vi "SW_Draw_mouse_DAQmx.vi"(0 "Image In":T1, 1 "Size of the image (480x480)":T3={"Numeric Control"=480.0, "Numeric Control"=480.0}, 5 "Pixels per mm":dbl=2.0, 7 "Mouse position":T2, 9 "Trace length, samples":u16=20 max=1000 step=1, 11 "Bright mouse lineout":bool=TRUE, 12 "Colors array input":u32[](array[colorbox]), 13 "Rainbow colors":bool=TRUE) -> (4 "Image Out":T1)   [LabVIEW 2018]
uses:
  <vilib>/vision/Image Controls.llb/IMAQ Image.ctl
  <vilib>/Utility/miscctls.llb/LVBoundsTypeDef.ctl
panel:
  in  "Experiment Diagram":T1(plugin-control)=refnum
  out "Time per draw":dbl
  in  "Trace color 2":u32(colorbox)
  in  "Trace color":u32(colorbox)=16757314
  in  "Mouse lineout color":u32(colorbox)=16775210
  in  "Iris size factor":dbl=0.05000000000000001 min=0.01 max=0.22 step=0.005 format="%#_13g"
  in  "Eye size factor":dbl=0.07000000000000002 min=0.02 max=0.24 step=0.01 format="%#_13g"
  out "Mouse abs. coordinates, pix":T3={"Numeric Control"=240.0, "Numeric Control"=240.0}
  in  "Mouse color":u32(colorbox)=5460819
  in  "Mouse length, mm":dbl=40.0
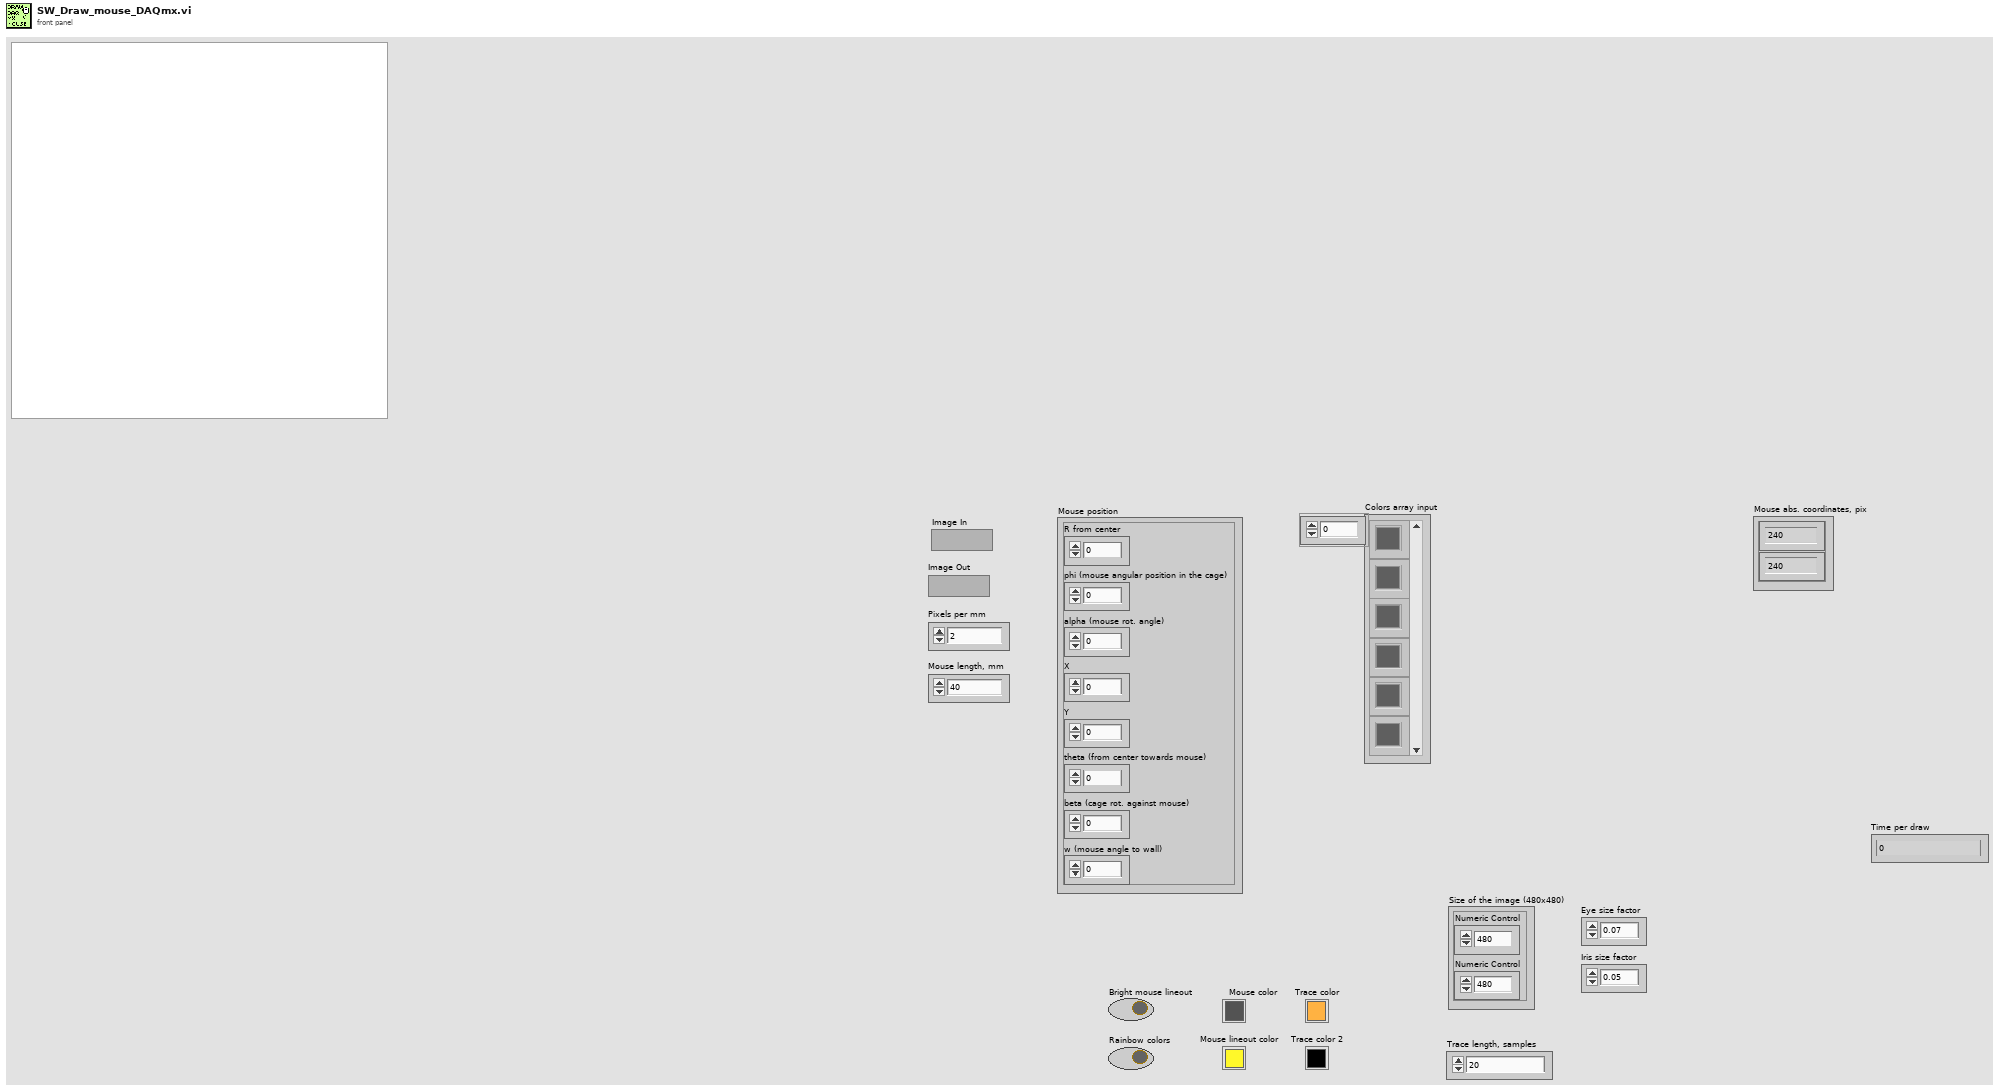
[diagram p1: front panel]
types:
  T1 = typedef "IMAQ Image.ctl" = refnum<image>
  T2 = cluster{"R from center":dbl, "phi (mouse angular position in the cage)":dbl, "alpha (mouse rot. angle)":sgl, "X":dbl, "Y":dbl, "theta (from center towards mouse)":dbl, "beta (cage rot. against mouse)":sgl, "w (mouse angle to wall)":dbl}
  T3 = cluster{"Numeric Control":dbl, "Numeric Control":dbl}
  T4 = cluster{"Width":u16, "Style":enum32{"Solid", "Dash", "Dot", "DashDot", "DashDotDot"}}
  T5 = typedef "LVBoundsTypeDef.ctl" = cluster{"Width":u32, "Height":u32}
  T6 = cluster{"Top":i32, "Left":i32, "Bottom":i32, "Right":i32}
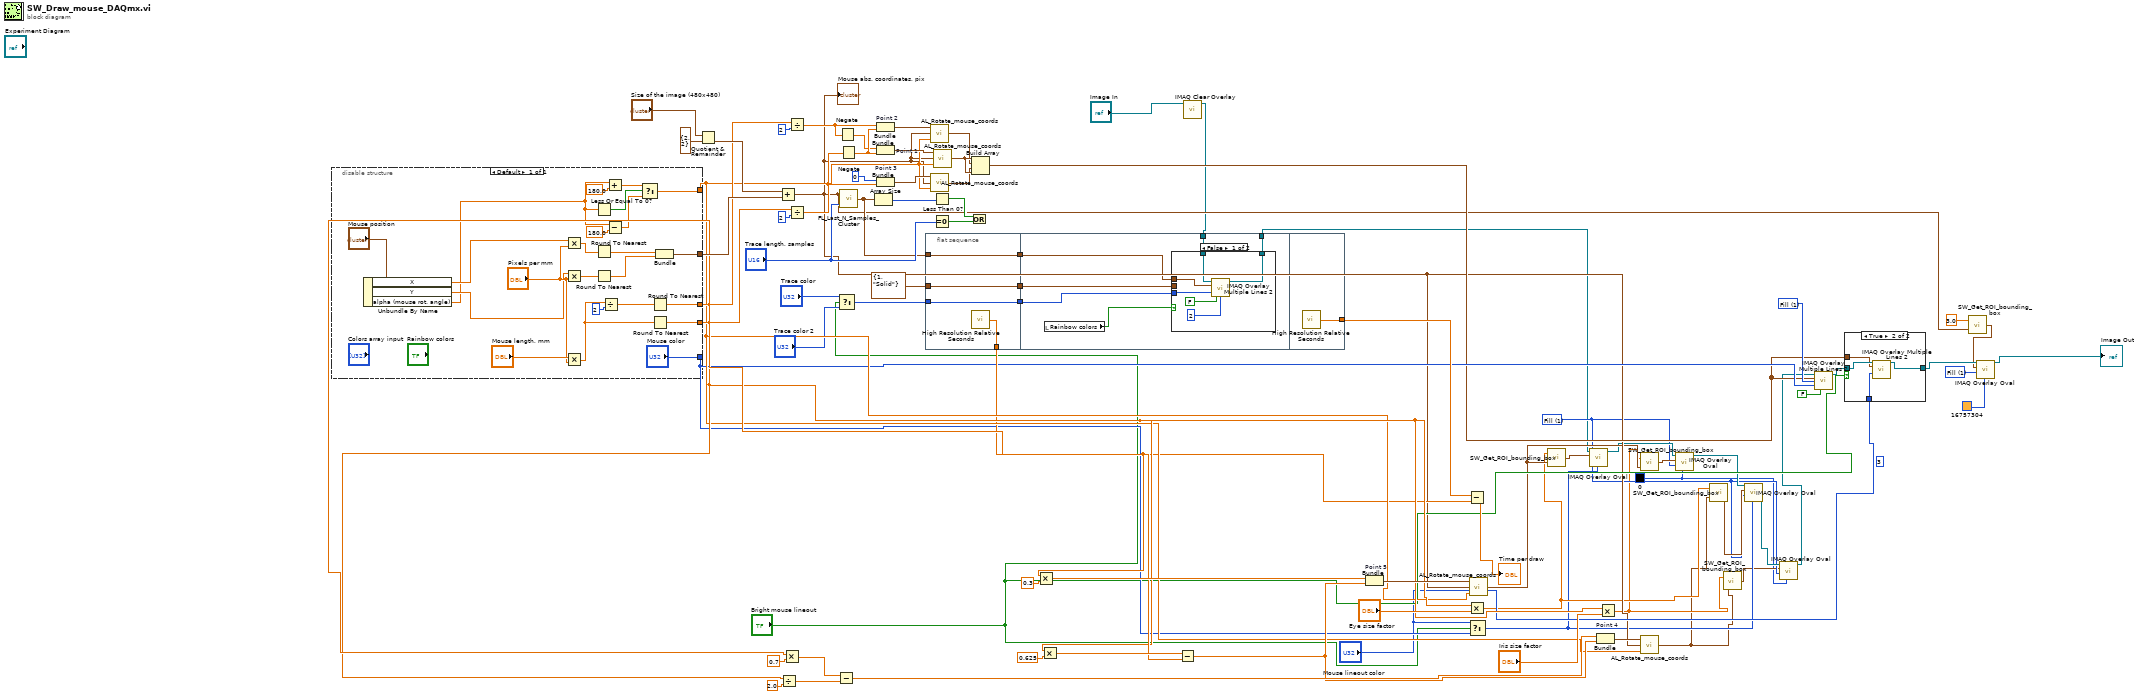
[diagram p0: block diagram]
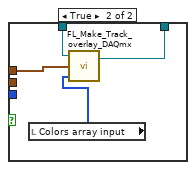
[diagram p3: hidden frame]
diagram:
  w4 = u32 0 ("Color")
  w8 = u32 1 items=["Frame", "Fill"] ("Drawing Mode (Frame)")
  w22 = u32 1 items=["Frame", "Fill"] ("Drawing Mode (Frame)")
  w32 = u32 1 items=["Frame", "Fill"] ("Drawing Mode (Frame)")
  (unwired) i16 3 ("radius")
  n1 = disable-structure shown="Default" {
    disable-tunnel: ["Mouse color"] -> w31
    disable-tunnel: [w98] -> w53
    disable-tunnel: [w100] -> w52
    disable-tunnel: [w86] -> w50
    disable-tunnel: [w92] -> w65
    frame Enabled {
      n2 = Unbundle By Name("Mouse position") -> ("X"=w84:dbl, "Y"=w83:dbl, "alpha (mouse rot. angle)"=w82:sgl)
      n3 = Multiply(x=w84, y="Pixels per mm") -> (x*y=w97:dbl)
      n4 = Multiply(x=w83, y="Pixels per mm") -> (x*y=w96:dbl)
      n5 = Multiply(x="Mouse length, mm", y="Pixels per mm") -> (x*y=w101:dbl)
      n6 = Less Or Equal To 0?(x=w82) -> (x <= 0?=w91:bool)
      n7 = Round To Nearest(number=w97) -> (nearest integer value=w94:dbl)
      n8 = Round To Nearest(number=w96) -> (nearest integer value=w93:dbl)
      n9 = Divide(x=w101, y=2) -> (x/y=w99:dbl)
      n10 = Add(x=w82, y=sgl 180.0) -> (x+y=w88:sgl)
      n11 = Subtract(x=w82, y=sgl 180.0) -> (x-y=w90:sgl)
      n12 = Select(t=w88, s=w91, f=w90) -> (s? t:f=w86:sgl)
      n13 = Round To Nearest(number=w99) -> (nearest integer value=w98:dbl)
      n14 = Round To Nearest(number=w101) -> (nearest integer value=w100:dbl)
      n15 = Bundle(w94, w93) -> (w92:cluster{dbl, dbl})  [unwired: 1 in]
    }
  }
  n16 = Quotient & Remainder(x="Size of the image (480x480)", y=T5 {"Width"=2, "Height"=2}) -> (floor(x/y)=w64:cluster{dbl, dbl})  [unwired: 1 out]
  n17 = Add(x=w64, y=w65) -> (x+y=w21:cluster{dbl, dbl})
  "Mouse abs. coordinates, pix" <- w21
  n18 = Divide(x=w52, y=2.0) -> (x/y=w58:dbl)
  n19 = Multiply(x=w53, y=0.7) -> (x*y=w62:dbl)
  n20 = Divide(x=w53, y=u16 2) -> (x/y=w49:dbl)
  n21 = Divide(x=w52, y=u16 2) -> (x/y=w78:dbl)
  n22 = Subtract(x=w62, y=w58) -> (x-y=w61:dbl)
  n23 = Select(t="Trace color", s="Bright mouse lineout", f="Trace color 2") -> (s? t:f=w42:u32)
  n24 = Negate(x=w49) -> (-x=w48:dbl)
  n25 = Negate(x=w78) -> (-x=w51:dbl)
  n26 = call "FL_Last_N_Samples_Cluster.vi"("BufferLengthSamples"="Trace length, samples", "Input cluster"=w21) -> ("Output 1D array of clusters"=w39:cluster{"X":dbl, "Y":dbl}[])
  n27 = Array Size(array=w39) -> (size(s)=w47:i32)
  n28 = Bundle "Point 2"(w49, w51) -> (w73:cluster{dbl, dbl})  [unwired: 1 in]
  n29 = Bundle "Point 1"(w48, w51) -> (w74:cluster{dbl, dbl})  [unwired: 1 in]
  n30 = Bundle "Point 3"(0, w78) -> (w72:cluster{i32, dbl})  [unwired: 1 in]
  n31 = flat-sequence {
    tunnel: w39 -> [w106]
    tunnel: T4 {"Width"=1, "Style"=enum."Solid"} ("pen") -> [w107]
    tunnel: w42 -> [w108]
    tunnel: [w108] -> w38
    tunnel: [w107] -> w37
    tunnel: [w106] -> w36
    tunnel: [w105] -> w34
    tunnel: w38 -> [w114]
    tunnel: w37 -> [w113]
    tunnel: w36 -> [w112]
    tunnel: w1 -> [w111]
    tunnel: [w110] -> w3
    tunnel: [w125] -> w35
    frame #0 {
      n32 = call <vilib>:"High Resolution Relative Seconds.vi"() -> ("relative seconds"=w105:dbl)
    }
    frame #1 {
      n33 = local read "Rainbow colors"() -> (w109:bool)
      n34 = case shown="False" w109 {
        tunnel: w114 -> [w118 _]
        tunnel: w113 -> [_ _]
        tunnel: w112 -> [w117 w124]
        tunnel: w111 -> [w120 w123]
        tunnel: [w119 w122] -> w110
        frame False {
          n35 = call "IMAQ Overlay Multiple Lines 2"("Image"=w120, "Line End Points"=w117, "Color"=w118, "Maintain Width?"=FALSE, "Width"=u32 2) -> ("Image Out"=w119:T1)  [unwired: 9 in, 1 out]
        }
        frame True {
          n36 = local read "Colors array input"() -> (w121:u32[])
          n37 = call "FL_Make_Track_overlay_DAQmx.vi"("Colors array input"=w121, "Full track array"=w124, "Image In"=w123) -> ("Image Out"=w122:T1)  [unwired: 2 in]
        }
      }
    }
    frame #2 {
      n38 = call <vilib>:"High Resolution Relative Seconds.vi"() -> ("relative seconds"=w125:dbl)
    }
  }
  n39 = call "AL_Rotate_mouse_coords.vi"("Mouse angle of rotation, deg"=w50, "Offset"=w21, "Coordinates to rotate"=w73) -> ("Rotated coordinates"=w68:cluster{"X":dbl, "Y":dbl})
  n40 = call "AL_Rotate_mouse_coords.vi"("Mouse angle of rotation, deg"=w50, "Offset"=w21, "Coordinates to rotate"=w72) -> ("Rotated coordinates"=w67:cluster{"X":dbl, "Y":dbl})
  n41 = call "AL_Rotate_mouse_coords.vi"("Mouse angle of rotation, deg"=w50, "Offset"=w21, "Coordinates to rotate"=w74) -> ("Rotated coordinates"=w69:cluster{"X":dbl, "Y":dbl})
  n42 = Less Than 0?(x=w47) -> (x < 0?=w45:bool)
  n43 = Equal To 0?(x="Trace length, samples") -> (x = 0?=w44:bool)
  n44 = Or(x=w45, y=w44) -> ()  [unwired: 1 out]
  n45 = Build Array(w69, w68, w67, w69) -> (w26:cluster{"X":dbl, "Y":dbl}[])
  n46 = Multiply(x=w53, y=0.3) -> (x*y=w56:dbl)
  n47 = Multiply(x=w52, y=0.625) -> (x*y=w59:dbl)
  n48 = Subtract(x=w59, y=w53) -> (x-y=w60:dbl)
  n49 = call "IMAQ Clear Overlay"("Image"="Image In") -> ("Image Out"=w1:T1)  [unwired: 9 in, 1 out]
  n50 = Bundle "Point 5"(w56, w60) -> (w70:cluster{dbl, dbl})  [unwired: 1 in]
  n51 = Subtract(x=w35, y=w34) -> (x-y=→"Time per draw":dbl)
  n52 = Multiply(x=w52, y="Eye size factor") -> (x*y=w14:dbl)
  n53 = Select(t="Mouse lineout color", s="Bright mouse lineout", f=w31) -> (s? t:f=w11:u32)
  n54 = call "AL_Rotate_mouse_coords.vi"("Mouse angle of rotation, deg"=w50, "Offset"=w21, "Coordinates to rotate"=w70) -> ("Rotated coordinates"=w17:cluster{"X":dbl, "Y":dbl})
  n55 = call "SW_Get_ROI_bounding_box.vi"("Center of the ROI"=w17, "Radius of the ROI, pix"=w14) -> ("Bounding box of the ROI, pix"=w18:T6)
  n56 = call "IMAQ Overlay Oval"("Color"=w11, "Drawing Mode (Frame)"=w8, "Bounding Rectangle"=w18, "Image"=w3) -> ("Image Out"=w15:T1)  [unwired: 6 in, 1 out]
  n57 = Bundle "Point 4"(w61, w60) -> (w71:cluster{dbl, dbl})  [unwired: 1 in]
  n58 = Multiply(x=w52, y="Iris size factor") -> (x*y=w7:dbl)
  n59 = call "SW_Get_ROI_bounding_box.vi"("Center of the ROI"=w17, "Radius of the ROI, pix"=w7) -> ("Bounding box of the ROI, pix"=w16:T6)
  n60 = call "AL_Rotate_mouse_coords.vi"("Mouse angle of rotation, deg"=w50, "Offset"=w21, "Coordinates to rotate"=w71) -> ("Rotated coordinates"=w6:cluster{"X":dbl, "Y":dbl})
  n61 = call "IMAQ Overlay Oval"("Color"=w4, "Drawing Mode (Frame)"=w8, "Bounding Rectangle"=w16, "Image"=w15) -> ("Image Out"=w13:T1)  [unwired: 6 in, 1 out]
  n62 = call "SW_Get_ROI_bounding_box.vi"("Center of the ROI"=w6, "Radius of the ROI, pix"=w14) -> ("Bounding box of the ROI, pix"=w12:T6)
  n63 = call "SW_Get_ROI_bounding_box.vi"("Center of the ROI"=w6, "Radius of the ROI, pix"=w7) -> ("Bounding box of the ROI, pix"=w5:T6)
  n64 = call "IMAQ Overlay Oval"("Color"=w11, "Drawing Mode (Frame)"=w8, "Bounding Rectangle"=w12, "Image"=w13) -> ("Image Out"=w10:T1)  [unwired: 6 in, 1 out]
  n65 = call "IMAQ Overlay Oval"("Color"=w4, "Drawing Mode (Frame)"=w8, "Bounding Rectangle"=w5, "Image"=w10) -> ("Image Out"=w9:T1)  [unwired: 6 in, 1 out]
  n66 = call "IMAQ Overlay Multiple Lines 2"("Image"=w9, "Line End Points"=w26, "Drawing Mode (Frame)"=w32, "Color"=w31, "Maintain Width?"=FALSE) -> ("Image Out"=w28:T1)  [unwired: 9 in, 1 out]
  n67 = case shown="True" "Bright mouse lineout" {
    tunnel: w28 -> [w126 w130]
    tunnel: [w126 w129] -> w25
    tunnel: "Mouse lineout color" -> [_ w128]
    tunnel: w26 -> [_ w127]
    frame False {
    }
    frame True {
      n68 = call "IMAQ Overlay Multiple Lines 2"("Image"=w130, "Line End Points"=w127, "Color"=w128) -> ("Image Out"=w129:T1)  [unwired: 11 in, 1 out]
    }
  }
  n69 = call "SW_Get_ROI_bounding_box.vi"("Center of the ROI"=w21, "Radius of the ROI, pix"=3.0) -> ("Bounding box of the ROI, pix"=w19:T6)
  n70 = call "IMAQ Overlay Oval"("Color"=u32 16757304 ("color(black)"), "Drawing Mode (Frame)"=w22, "Bounding Rectangle"=w19, "Image"=w25) -> ("Image Out"=→"Image Out":T1)  [unwired: 6 in, 1 out]
